vi "FTW-Endpoint-Bind.vi"(0 "FTW Endpoint":refnum<class "FTW-Endpoint-Notifier.lvclass">, 5 "Endpoint Address":string, 7 "Requested Identity":string, 11 "error in":errorcluster) -> (4 "FTW Endpoint out":refnum<class "FTW-Endpoint-Notifier.lvclass">, 6 "Actual Endpoint Address":string, 8 "Actual Identity":string, 15 "error out":errorcluster)   [LabVIEW 2013, in "FTW-Endpoint-Notifier.lvclass"]
uses:
  FTW-Endpoint-Notifier.lvclass
  FTW-Endpoint-Notifier.lvclass/FTW-Endpoint-Notifier.ctl
panel:
  # "Inputs"
  # "Outputs"
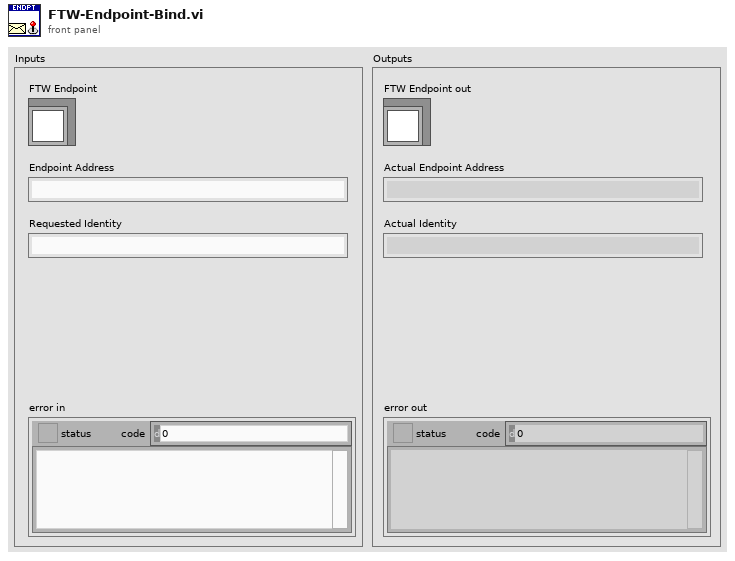
[diagram p1: front panel]
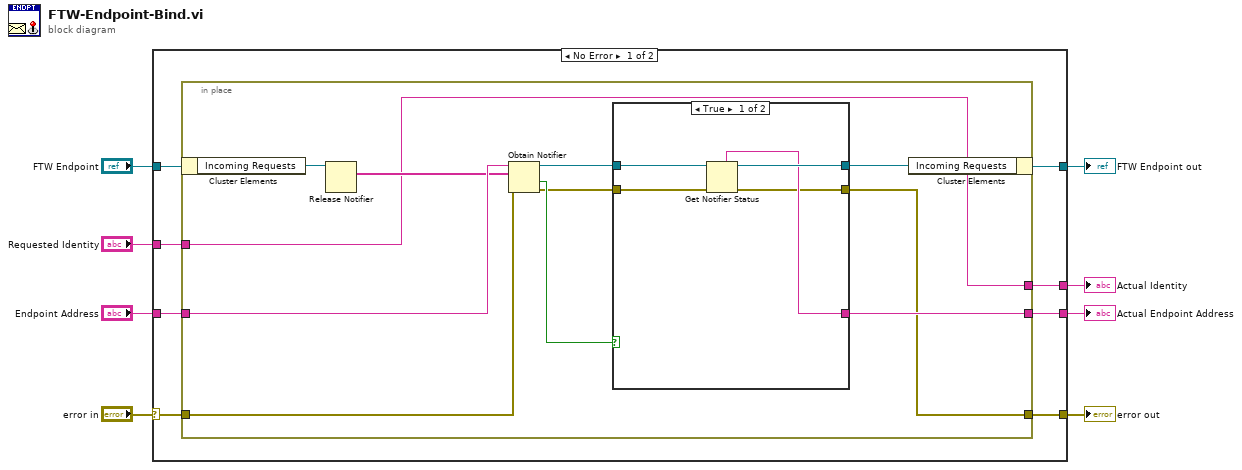
[diagram p0: block diagram]
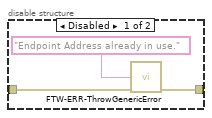
[diagram p3: hidden frame]
diagram:
  n1 = case shown="No Error" "error in" {
    selector: "error in" -> [w14 w41]
    tunnel: [w10 w41] -> w8
    tunnel: [w11 w40] -> w6
    tunnel: "FTW Endpoint" -> [w16 w40]
    tunnel: "Requested Identity" -> [w15 _]
    tunnel: "Endpoint Address" -> [w13 _]
    tunnel: [w12 _] -> w2
    tunnel: [w9 _] -> w1
    frame No Error {
      n2 = in-place {
        in-place-border: w15 -> [w17]
        in-place-border: w14 -> [w26]
        in-place-border: [w19] -> w10
        in-place-border: w13 -> [w23]
        in-place-border: [w24] -> w12
        in-place-border: [w17] -> w9
        n3 = in-place-cluster #1(w16) -> ("Incoming Requests"=w27:refnum<notifier>)
        n4 = Release Notifier(notifier=w27) -> (last notification=w18:string[])  [unwired: 2 in, 2 out]
        n5 = Obtain Notifier(name (unnamed)=w23, notification data type=w18, error in (no error)=w26) -> (notifier out=w21:refnum<notifier>, created new?=w25:bool, error out=w20:errorcluster)  [unwired: 1 in]
        n6 = case shown="True" w25 {
          tunnel: [w29 _] -> w24
          tunnel: [w31 w34] -> w22
          tunnel: w21 -> [w32 w34]
          tunnel: w20 -> [w30 w35]
          tunnel: [w28 w33] -> w19
          frame True {
            n7 = Get Notifier Status(notifier=w32, error in (no error)=w30) -> (notifier out=w31:refnum<notifier>, notifier name=w29:string, error out=w28:errorcluster)  [unwired: 2 out]
          }
          frame False {
            n8 = disable-structure shown="Enabled" {
              disable-tunnel: w35 -> [w38 w39]
              disable-tunnel: [w37 w39] -> w33
              frame Disabled {
                n9 = call "FTW-ERR-ThrowGenericError.vi"("Error Message"="Endpoint Address already in use.", "error in"=w38) -> ("error out"=w37:errorcluster)  [unwired: 13 in]
              }
              frame Enabled {
              }
            }
          }
        }
        n10 = in-place-cluster #1("Incoming Requests"=w22) -> (w11:refnum<class "FTW-Endpoint-Notifier.lvclass">)
      }
    }
    frame Error {
    }
  }
  "error out" <- w8
  "FTW Endpoint out" <- w6
  "Actual Endpoint Address" <- w2
  "Actual Identity" <- w1
